vi "Read Excel file.vi"(1 "Array":path[](array[path]), 2 "Start and End":T1) -> (0 "array":dbl[][][](array[numeric]))   [LabVIEW 2014]
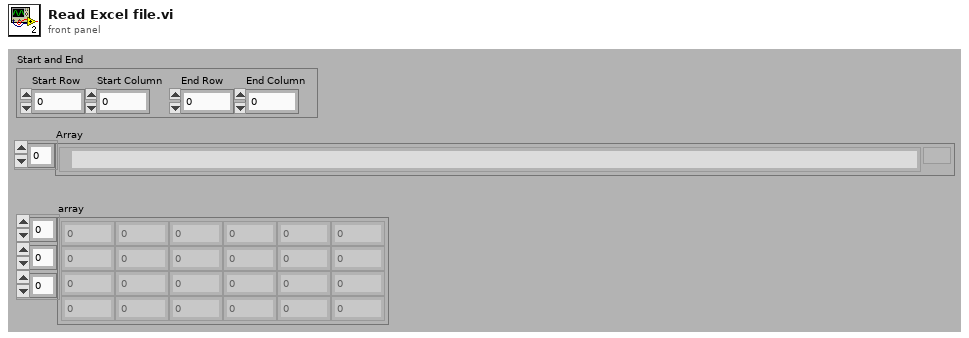
[diagram p1: front panel]
types:
  T1 = cluster{"Start Row":i32, "Start Column":i32, "End Row":i32, "End Column":i32}
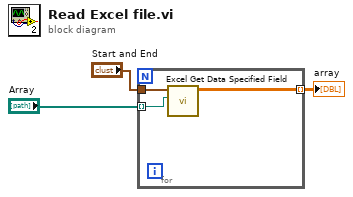
[diagram p0: block diagram]
diagram:
  n1 = for {
    tunnel: "Start and End" -> [w6]
    tunnel: "Array" -> [w5] mode=indexing
    tunnel: [w4] -> w1 mode=indexing
    n2 = call "Excel Get Data Specified Field.vi"("path"=w5, "Start and End"=w6) -> ("array"=w4:dbl[][])  [unwired: 3 in, 2 out]
  }
  "array" <- w1
